vi "Timer Count 3 with Error Handling.vi"(6 "Reset":bool, 8 "error in (no error)":errorcluster, 11 "Timeout (ms)":u32) -> (0 "error out":errorcluster, 1 "Time(s)":dbl, 2 "Time (ms)":u32, 3 "Time(min)":dbl, 4 "Timer Elapsed?":bool)   [LabVIEW 2014, in "Utilities.lvlib"]
uses:
  Utilities.lvlib
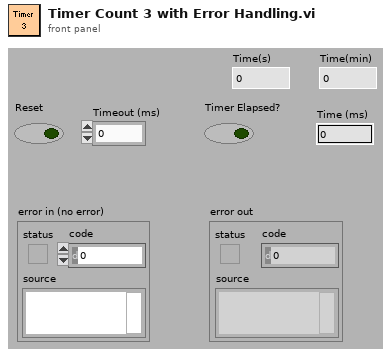
[diagram p1: front panel]
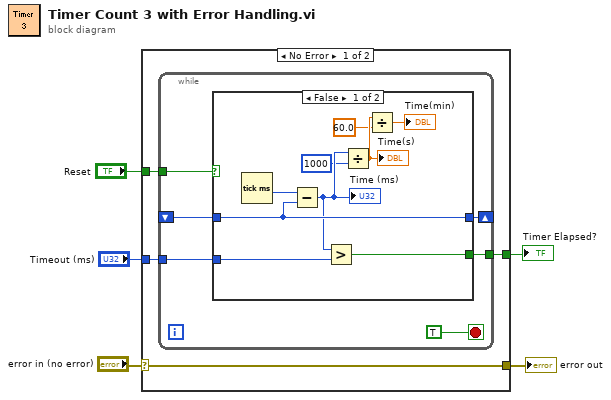
[diagram p0: block diagram]
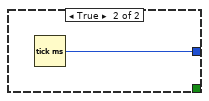
[diagram p2: hidden frame]
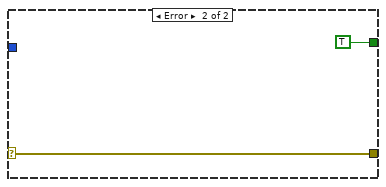
[diagram p3: hidden frame]
diagram:
  n1 = case shown="No Error" "error in (no error)" {
    selector: "error in (no error)" -> [w9 w27]
    tunnel: [w9 w27] -> w4
    tunnel: "Reset" -> [w8 _]
    tunnel: "Timeout (ms)" -> [w7 _]
    tunnel: [w6 TRUE] -> w1
    frame No Error {
      n2 = while {
        shift-right: [w14] -> _
        shift-left: _ -> [w12]
        tunnel: w8 -> [w13]
        tunnel: w7 -> [w11]
        tunnel: [w10] -> w6
        stop <- TRUE stop-if-true
        n3 = case shown="False" w13 {
          tunnel: [w23 w25] -> w14
          tunnel: w12 -> [w23 _]
          tunnel: w11 -> [w22 _]
          tunnel: [w21 _] -> w10
          frame False {
            n4 = Tick Count (ms)() -> (millisecond timer value=w24:u32)
            n5 = Subtract(x=w24, y=w23) -> (x-y=w20:u32)
            "Time (ms)" <- w20
            n6 = Greater?(x=w20, y=w22) -> (0:w21:bool)
            n7 = Divide(x=w20, y=u32 1000) -> (x/y=w18:dbl)
            "Time(s)" <- w18
            n8 = Divide(x=w18, y=60.0) -> (x/y=→"Time(min)":dbl)
          }
          frame True {
            n9 = Tick Count (ms)() -> (millisecond timer value=w25:u32)
          }
        }
      }
    }
    frame Error {
    }
  }
  "error out" <- w4
  "Timer Elapsed?" <- w1
